vi "IsRefnum.vi"(8 "error in":errorcluster, 11 "CustomElement in":refnum<class "CustomElement.lvclass">) -> (0 "error out":errorcluster, 2 "IsRefnum":bool, 3 "CustomElement out":refnum<class "CustomElement.lvclass">)   [LabVIEW 2021, in "ProligentXMLGenerator.lvlib" / "CustomElement.lvclass"]
doc: "Returns TRUE if the passed object is valid."
uses:
  CustomElement.lvclass
  CustomElement.lvclass/CustomElement.ctl
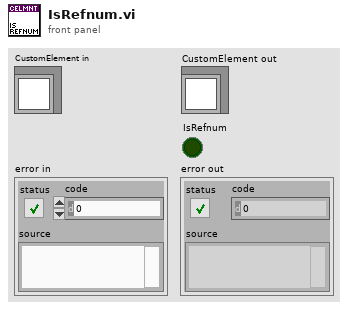
[diagram p1: front panel]
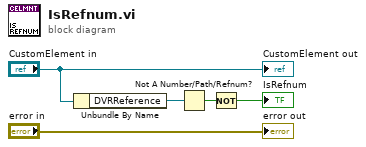
[diagram p0: block diagram]
diagram:
  n1 = Unbundle By Name("CustomElement in") -> ("DVRReference"=w1:refnum<data-value>)
  n2 = Not A Number/Path/Refnum?(number/path/refnum=w1) -> (NaN/Path/Refnum?=w3:bool)
  n3 = Not(x=w3) -> (.not. x?=→"IsRefnum":bool)
  "error out" <- "error in"
  "CustomElement out" <- "CustomElement in"
